vi "Set Global Broadcast Filter.vi"(10 "Group:Broadcast":string[](array[string]), 11 "GlobalLogFilter In":refnum<class "LogFilter.lvclass">) -> (3 "GlobalLogFilter Out":refnum<class "LogFilter.lvclass">)   [LabVIEW 2017, in "Communicable State Machine.lvlib" / "LogFilter.lvclass"]
doc: "### Set Global State Filter.vi\n\n-- <b>Controls</b> --\n- <b>Group:State</b>:\n- <b>GlobalLogFilter in</b>:\n\n-- <b>Indicators</b> --\n- <b>GlobalLogFilter out</b>:"
uses:
  LogFilter.lvclass
  LogFilter.lvclass/LogFilter.ctl
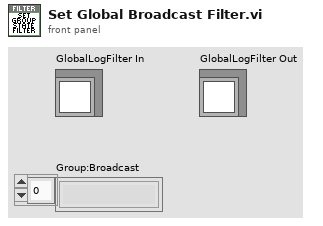
[diagram p1: front panel]
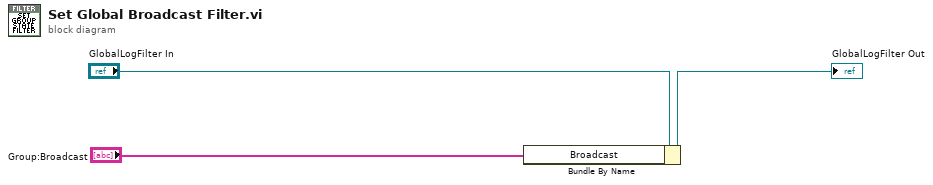
[diagram p0: block diagram]
diagram:
  n1 = Bundle By Name(cluster="GlobalLogFilter In", "Broadcast"="Group:Broadcast") -> (→"GlobalLogFilter Out":refnum<class "LogFilter.lvclass">)
